vi "UHR-Fleezers Control (host) - 12.0_test_fpga_connection.vi"() -> ()   [LabVIEW 2014] (continued)
                n3308 = local read "N sets should be saved (MCL)"() -> (w5191:dbl)
                n3309 = Build Array(w5188, w5180, w5182, w5182, w5182) -> (w5186:dbl[])
                n3310 = Build Array(w5203, w5198, w5196, w5194, w5193, w5184, w5183) -> (w5200:dbl[])
                n3311 = Build Array(w5185, w5189, w5209, w5208, w5207, 3.0 ("t")) -> (w5202:dbl[])
                n3312 = Round Toward +Infinity(x=w5191) -> (ceil(x): smallest int >= x=w5192:dbl)
                n3313 = Build Array (concatenate)(w5202, w5201, w5186, w5200) -> (w5199:dbl[])
                n3314 = To Unsigned Long Integer(number=w5192) -> (unsigned 32bit integer=w5190:u32)
              }
            }
            n3315 = local read "Index"() -> (w5045:dbl)
            n3316 = call "Create new save file.vi"("Insert"="", "Ext"=".dat", "Index In"=w5045) -> ("Path Out"=w5004:path, "Index Out"=w5017:dbl)
            n3317 = local write "Save file name"(w5004) -> ()
            n3318 = local write "Index"(w5017) -> ()
            n3319 = local write "Save index"(w5017) -> ()
            n3320 = Array Size(array=w5028) -> (size(s)=w5029:i32)
            n3321 = Open/Create/Replace File(file path (use dialog)=w5004, operation (0:open)=T30."create", access (0:read/write)=enum16{"read/write", "read-only", "write-only"}."write-only") -> (refnum out=w5042:refnum<file>)  [unwired: 1 in, 4 out]
            n3322 = local write "Saving..."(TRUE ("Saving...")) -> ()
            n3323 = To Double Precision Float(number=w5029) -> (double precision float=w5027:dbl)
            n3324 = String Length(string="Comment (data description)") -> (length=w5025:i32)
            n3325 = To Double Precision Float(number=w5025) -> (double precision float=w5024:dbl)
            n3326 = Deny Access(7:w5042) -> (3:w5041:refnum<file>)  [unwired: 1 in, 2 out]
            n3327 = Build Array (concatenate)(w5027, w5028, w5024) -> (w5026:dbl[])
            n3328 = case "If fluorescence data to be saved" shown="True" w5015 {
              tunnel: w5004 -> [_ w5094]
              tunnel: [refnum<k0> refnum w5074] -> w5016
              frame False {
              }
              frame True {
                w5073 = 0.0
                n3329 = local read "APD Integration Time (s)"() -> (w5079:dbl)
                n3330 = local read "N APD Samp/step"() -> (w5072:dbl)
                n3331 = Path To String(path=w5094) -> (string=w5093:string)
                n3332 = String Length(string=w5093) -> (length=w5092:i32)
                n3333 = Subtract(x=w5092, y=4) -> (x-y=w5090:i32)
                n3334 = String Subset(string=w5093, length (rest)=w5090) -> (substring=w5089:string)  [unwired: 1 out]
                n3335 = Build Array(w5079, w5072, w5073, w5073, w5073, w5073, w5073, w5073) -> (w5076:dbl[])
                n3336 = Concatenate Strings(w5089, "_fl.dat" ("string")) -> (w5087:string)
                n3337 = Array Size(array=w5076) -> (size(s)=w5078:i32)
                n3338 = String To Path(string=w5087) -> (path=w5083:path)
                n3339 = Open/Create/Replace File(file path (use dialog)=w5083, operation (0:open)=T30."create", access (0:read/write)=enum16{"read/write", "read-only", "write-only"}."write-only") -> (refnum out=w5084:refnum<file>)  [unwired: 1 in, 4 out]
                n3340 = Deny Access(7:w5084) -> (3:w5080:refnum<file>)  [unwired: 1 in, 2 out]
                n3341 = To Double Precision Float(number=w5078) -> (double precision float=w5077:dbl)
                n3342 = Build Array (concatenate)(w5077, w5076) -> (w5075:dbl[])
                n3343 = Write to Binary File(file (use dialog)=w5080, data=w5075, 5:FALSE ("prepend array or string size? (T)"), 9:T29."big-endian, network order" ("byte order (0:big-endian, network order)")) -> (refnum out=w5074:refnum<file>)  [unwired: 1 in, 3 out]
              }
            }
            n3344 = case shown="True" w5002 {
              tunnel: w5004 -> [_ w5056]
              tunnel: [refnum<k0> refnum w5055] -> w5003
              frame False {
              }
              frame True {
                w5051 = 0.0 ("element")
                n3345 = Path To String(path=w5056) -> (string=w5070:string)
                n3346 = Build Array(w5051, w5051, w5051, w5051, w5051, w5051, w5051, w5051) -> (w5052:dbl[])
                n3347 = String Length(string=w5070) -> (length=w5069:i32)
                n3348 = Subtract(x=w5069, y=4) -> (x-y=w5067:i32)
                n3349 = Array Size(array=w5052) -> (size(s)=w5054:i32)
                n3350 = String Subset(string=w5070, length (rest)=w5067) -> (substring=w5066:string)  [unwired: 1 out]
                n3351 = To Double Precision Float(number=w5054) -> (double precision float=w5053:dbl)
                n3352 = Concatenate Strings(w5066, "_pos.dat" ("string")) -> (w5064:string)
                n3353 = Build Array (concatenate)(w5053, w5052) -> (w5050:dbl[])
                n3354 = String To Path(string=w5064) -> (path=w5060:path)
                n3355 = Open/Create/Replace File(file path (use dialog)=w5060, operation (0:open)=T30."create", access (0:read/write)=enum16{"read/write", "read-only", "write-only"}."write-only") -> (refnum out=w5061:refnum<file>)  [unwired: 1 in, 4 out]
                n3356 = Deny Access(7:w5061) -> (3:w5057:refnum<file>)  [unwired: 1 in, 2 out]
                n3357 = Write to Binary File(file (use dialog)=w5057, data=w5050, 5:FALSE ("prepend array or string size? (T)"), 9:T29."big-endian, network order" ("byte order (0:big-endian, network order)")) -> (refnum out=w5055:refnum<file>)  [unwired: 1 in, 3 out]
              }
            }
            n3358 = Write to Binary File(file (use dialog)=w5041, data=w5026, 5:w5022, 9:w5020) -> (refnum out=w5023:refnum<file>)  [unwired: 1 in, 3 out]
            n3359 = Write to Binary File(file (use dialog)=w5023, data="Comment (data description)", 5:w5022, 9:w5020) -> (refnum out=w5019:refnum<file>)  [unwired: 1 in, 3 out]
          }
        }
        n3360 = feedback-in #32(w4963) -> ()
        n3361 = feedback-in #33(w4989) -> ()
        n3362 = feedback-in #34(w4962) -> ()
        n3363 = feedback-in #35(w4973) -> ()
        n3364 = feedback-in #36(w4976) -> ()
        n3365 = feedback-in #37(w4988) -> ()
        n3366 = feedback-in #38(w4979) -> ()
      }
      frame #1 {
        n3367 = local read "Saving..."() -> (w5224:bool)
        n3368 = case shown="True" w5224 {
          tunnel: w5228 -> [_ w5240]
          tunnel: w5227 -> [_ w5253]
          tunnel: w5226 -> [_ w5249]
          tunnel: w5225 -> [_ w5248]
          tunnel: w5223 -> [_ w5229]
          tunnel: w5222 -> [_ w5243]
          tunnel: w5221 -> [_ w5242]
          tunnel: w5220 -> [_ w5241]
          tunnel: w5219 -> [_ w5239]
          tunnel: w5218 -> [_ w5237]
          tunnel: w5217 -> [_ w5236]
          tunnel: w5216 -> [_ w5235]
          tunnel: w5215 -> [_ w5234]
          tunnel: w5214 -> [_ w5233]
          tunnel: w5213 -> [_ w5232]
          tunnel: w5212 -> [_ w5231]
          tunnel: w5211 -> [_ w5230]
          frame False {
          }
          frame True {
            n3369 = Multiply(x=w5240, y=w5239) -> (x*y=→"Time (s)":dbl)
            n3370 = Less Or Equal?(x=w5240, y=w5229) -> (x <= y?=w5251:bool)
            n3371 = Or(x="Stop Saving", y="Abort save 2") -> (x .or. y?=w5244:bool)
            n3372 = Not(x=w5244) -> (.not. x?=w5252:bool)
            n3373 = And(x=w5251, y=w5252) -> (x .and. y?=w5250:bool)
            n3374 = case shown="True" w5250 {
              tunnel: w5253 -> [w5261 w5336]
              tunnel: [0.0 w5339] -> w5247
              tunnel: w5240 -> [_ w5337]
              tunnel: w5229 -> [_ w5338]
              tunnel: w5249 -> [_ w5333]
              tunnel: w5248 -> [_ _]
              tunnel: w5243 -> [w5259 w5326]
              tunnel: w5242 -> [w5258 w5327]
              tunnel: w5241 -> [_ w5325]
              tunnel: w5237 -> [_ w5324]
              tunnel: w5236 -> [_ w5268]
              tunnel: w5235 -> [_ w5317]
              tunnel: w5234 -> [_ w5295]
              tunnel: w5233 -> [w5255 w5277]
              tunnel: w5232 -> [w5256 w5276]
              tunnel: w5231 -> [_ w5273]
              tunnel: w5230 -> [_ w5271]
              frame False {
                w5257 = FALSE
                n3375 = Close File(refnum=w5261) -> ()  [unwired: 1 in, 2 out]
                n3376 = case shown="True" w5258 {
                  tunnel: w5259 -> [_ w5263]
                  frame False {
                  }
                  frame True {
                    n3377 = Close File(refnum=w5263) -> ()  [unwired: 1 in, 2 out]
                  }
                }
                n3378 = case shown="True" w5255 {
                  tunnel: w5256 -> [_ w5262]
                  frame False {
                  }
                  frame True {
                    n3379 = Close File(refnum=w5262) -> ()  [unwired: 1 in, 2 out]
                  }
                }
                n3380 = call <vilib>:"Beep.vi"() -> ()  [unwired: 3 in, 9 out]
                n3381 = local write "Raster Scanning..."(w5257) -> ()
                n3382 = local write "Calibrating..."(w5257) -> ()
                n3383 = property on="Abort wiggle" class="Bool (strict)"("Val(Sgnl)"=TRUE) -> ()  [unwired: 2 in, 2 out]
                n3384 = local write "Stop Saving"(w5257) -> ()
                "Saving..." <- w5257
              }
              frame True {
                n3385 = local read "Calibrating..."() -> (w5328:bool)
                n3386 = case "Write fl. data" shown="True" w5327 {
                  tunnel: w5326 -> [_ w5362]
                  tunnel: w5325 -> [_ w5361]
                  frame False {
                  }
                  frame True {
                    n3387 = Write to Binary File(file (use dialog)=w5362, data=w5361, 5:FALSE ("prepend array or string size? (T)"), 9:T29."big-endian, network order" ("byte order (0:big-endian, network order)")) -> ()  [unwired: 1 in, 4 out]
                  }
                }
                n3388 = Greater?(x="Save ave N", y=1.0) -> (0:w5331:bool)
                n3389 = Not(x=w5328) -> (.not. x?=w5330:bool)
                n3390 = And(x=w5330, y=w5331) -> (x .and. y?=w5274:bool)
                n3391 = case shown="True" w5274 {
                  tunnel: w5273 -> [w5342 w5353]
                  tunnel: [w5342 w5345] -> w5272
                  tunnel: "Save ave N" -> [_ w5346]
                  frame False {
                  }
                  frame True {
                    w5343 = 2 ("dimension size")
                    n3392 = Array Size(array=w5353) -> (size(s)=w5347:i32)
                    n3393 = Divide(x=w5347, y=w5343) -> (x/y=w5351:dbl)
                    n3394 = Reshape Array(w5353, w5351, w5343) -> (w5352:u64[][])
                    n3395 = Transpose 2D Array(2D array=w5352) -> (transposed array=w5350:u64[][])
                    n3396 = for {
                      tunnel: w5350 -> [w5355] mode=indexing
                      tunnel: [w5354] -> w5344 mode=indexing
                      tunnel: w5346 -> [w5356]
                      workers-P: _ -> [_]
                      n3397 = call "downsample 1D array - U64.vi"("Ave N"=w5356, "Array In"=w5355) -> ("Array Out"=w5354:u64[])  [unwired: 1 in]
                    }
                    n3398 = Transpose 2D Array(2D array=w5344) -> (transposed array=w5349:u64[][])
                    n3399 = Divide(x=w5347, y=w5346) -> (x/y=w5348:dbl)
                    n3400 = Reshape Array(w5349, w5348) -> (w5345:u64[])
                  }
                }
                n3401 = case shown="True" w5274 {
                  tunnel: w5333 -> [w5365 w5377]
                  tunnel: [w5365 w5369] -> w5329
                  tunnel: "Save ave N" -> [_ w5370]
                  tunnel: w5324 -> [_ w5368]
                  frame False {
                  }
                  frame True {
                    n3402 = Array Size(array=w5377) -> (size(s)=w5371:i32)
                    n3403 = Array Size(array=w5368) -> (size(s)=w5367:i32)
                    n3404 = Divide(x=w5371, y=w5367) -> (x/y=w5375:dbl)
                    n3405 = Reshape Array(w5377, w5375, w5367) -> (w5376:i16[][])
                    n3406 = Transpose 2D Array(2D array=w5376) -> (transposed array=w5374:i16[][])
                    n3407 = for {
                      tunnel: w5374 -> [w5380] mode=indexing
                      tunnel: [w5379] -> w5366 mode=indexing
                      tunnel: w5370 -> [w5378]
                      workers-P: _ -> [_]
                      n3408 = call "downsample 1D array - I16.vi"("Ave N"=w5378, "Array In"=w5380) -> ("Array Out"=w5379:i16[])  [unwired: 1 out]
                    }
                    n3409 = Transpose 2D Array(2D array=w5366) -> (transposed array=w5373:i16[][])
                    n3410 = Divide(x=w5371, y=w5370) -> (x/y=w5372:dbl)
                    n3411 = Reshape Array(w5373, w5372) -> (w5369:i16[])
                  }
                }
                n3412 = Index Array(array=w5295, index=1) -> (element=w5298:waveform(dbl))
                n3413 = Index Array(array=w5295, index=0) -> (element=w5300:waveform(dbl))
                n3414 = Unbundle By Name(w5298) -> ("Y"=w5302:dbl[])
                n3415 = Unbundle By Name(w5300) -> ("Y"=w5310:dbl[])
                n3416 = case "Write trap pos. data" shown="True" w5277 {
                  tunnel: w5276 -> [_ w5358]
                  tunnel: w5272 -> [_ w5357]
                  frame False {
                  }
                  frame True {
                    n3417 = Write to Binary File(file (use dialog)=w5358, data=w5357, 5:FALSE ("prepend array or string size? (T)"), 9:T29."big-endian, network order" ("byte order (0:big-endian, network order)")) -> ()  [unwired: 1 in, 4 out]
                  }
                }
                n3418 = Write to Binary File(file (use dialog)=w5336, data=w5329, 5:FALSE ("prepend array or string size? (T)"), 9:T29."big-endian, network order" ("byte order (0:big-endian, network order)")) -> ()  [unwired: 1 in, 4 out]
                n3419 = feedback #39(w5302) -> (w5304:dbl[])
                n3420 = Build Array (concatenate)(w5304, w5302) -> (w5303:dbl[])
                n3421 = Select(t=w5302, s=w5268, f=w5303) -> (s? t:f=w5288:dbl[])
                n3422 = feedback-in #39(w5288) -> ()
                n3423 = feedback #40(w5310) -> (w5323:dbl[])
                n3424 = Build Array (concatenate)(w5323, w5310) -> (w5322:dbl[])
                n3425 = Select(t=w5310, s=w5268, f=w5322) -> (s? t:f=w5297:dbl[])
                n3426 = feedback-in #40(w5297) -> ()
                n3427 = Divide(x=w5337, y=w5338) -> (x/y=w5340:dbl)
                n3428 = Multiply(x=w5340, y=100.0) -> (x*y=w5339:dbl)
                n3429 = Build Array(w5297, w5288) -> (→"Saved APD":dbl[][])
                n3430 = Array Size(array=w5297) -> (size(s)=w5315:i32)
                n3431 = Unbundle By Name(w5317) -> ("Y"=w5321:dbl[])
                n3432 = Subtract(x=w5315, y="N pts to average") -> (x-y=w5291:i32)
                n3433 = Multiply(x="N pts to average", y=u16 2) -> (x*y=w5292:u16)
                n3434 = Subtract(x=w5315, y=w5292) -> (x-y=w5290:i32)
                n3435 = feedback #41(w5321) -> (w5320:dbl[])
                n3436 = Build Array (concatenate)(w5320, w5321) -> (w5319:dbl[])
                n3437 = Select(t=w5321, s=w5268, f=w5319) -> (s? t:f=w5318:dbl[])
                "Trap Delta Graph" <- w5318
                n3438 = feedback-in #41(w5318) -> ()
                n3439 = Array Subset(array=w5297, index=w5291, length="N pts to average") -> (w5314:dbl[])
                n3440 = Array Subset(array=w5297, index=w5290, length="N pts to average") -> (w5313:dbl[])
                n3441 = Array Subset(array=w5288, index=w5291, length="N pts to average") -> (w5294:dbl[])
                n3442 = Array Subset(array=w5288, index=w5290, length="N pts to average") -> (w5293:dbl[])
                n3443 = Index Array(array=w5271, index=0) -> (element=w5269:waveform(dbl))
                n3444 = call-poly <vilib>:"Mean.vi"("X"=w5314) -> ("mean"=w5312:dbl)  [unwired: 1 out]
                n3445 = call-poly <vilib>:"Mean.vi"("X"=w5294) -> ("mean"=w5287:dbl)  [unwired: 1 out]
                n3446 = call-poly <vilib>:"Mean.vi"("X"=w5313) -> ("mean"=w5311:dbl)  [unwired: 1 out]
                n3447 = call-poly <vilib>:"Mean.vi"("X"=w5293) -> ("mean"=w5286:dbl)  [unwired: 1 out]
                n3448 = Unbundle By Name(w5269) -> ("Y"=w5266:dbl[])
                n3449 = Subtract(x=w5287, y=w5286) -> (x-y=w5278:dbl)
                "Delta Fl. 2" <- w5278
                n3450 = Subtract(x=w5312, y=w5311) -> (x-y=w5309:dbl)
                "Delta Fl. 1" <- w5309
                n3451 = Initialize Array(w5309, 1 ("dimension size")) -> (w5306:dbl[])
                n3452 = Initialize Array(w5278, 1 ("dimension size")) -> (w5283:dbl[])
                n3453 = feedback #42(w5306) -> (w5307:dbl[])
                n3454 = Build Array (concatenate)(w5307, w5306) -> (w5305:dbl[])
                n3455 = feedback #43(w5283) -> (w5284:dbl[])
                n3456 = Build Array (concatenate)(w5284, w5283) -> (w5282:dbl[])
                n3457 = feedback #44(w5266) -> (w5265:dbl[])
                n3458 = Build Array (concatenate)(w5265, w5266) -> (w5267:dbl[])
                n3459 = Select(t=w5266, s=w5268, f=w5267) -> (s? t:f=w5264:dbl[])
                "Saved trap pos" <- w5264
                n3460 = feedback-in #44(w5264) -> ()
                n3461 = Select(t=w5306, s=w5268, f=w5305) -> (s? t:f=w5281:dbl[])
                n3462 = feedback-in #42(w5281) -> ()
                n3463 = Select(t=w5283, s=w5268, f=w5282) -> (s? t:f=w5280:dbl[])
                n3464 = feedback-in #43(w5280) -> ()
                n3465 = Build Array(w5281, w5280) -> (→"Save APD Deriv":dbl[][])
              }
            }
            "Progress" <- w5247
            "Progress 2" <- w5247
          }
        }
      }
    }
    n3466 = local read "wait to reset values"() -> (w3911:bool)
    n3467 = Not(x=w3909) -> (.not. x?=w3912:bool)
    n3468 = And(x=w3912, y=w3911) -> (x .and. y?=w3913:bool)
    n3469 = case "Part of MCL raster scanning: returns to initial positions after scan done" shown="True" w3913 {
      tunnel: w3654 -> [w4782 w4789]
      tunnel: [w4782 w4788] -> w3915
      tunnel: w3653 -> [w4781 w4787]
      tunnel: [w4781 w4786] -> w3910
      frame False {
      }
      frame True {
        w4797 = 10.0 ("y")
        w4796 = 32767.0 ("y")
        # "to return scan values\nafter a synchronous \nAOM scan"
        n3470 = local read "AO2"() -> (w4790:dbl)
        n3471 = local read "AO1"() -> (w4791:dbl)
        n3472 = local write "wait to reset values"(FALSE ("wait to reset values")) -> ()
        n3473 = Multiply(x=w4791, y=w4796) -> (x*y=w4793:dbl)
        n3474 = Multiply(x=w4790, y=w4796) -> (x*y=w4795:dbl)
        n3475 = Divide(x=w4793, y=w4797) -> (x/y=w4792:dbl)
        n3476 = Divide(x=w4795, y=w4797) -> (x/y=w4794:dbl)
        n3477 = To Word Integer(number=w4792) -> (16bit integer=w4798:i16)
        n3478 = To Word Integer(number=w4794) -> (16bit integer=w4799:i16)
        n3479 = local read "Total Counts (ticks)"() -> (w4783:u32)
        n3480 = xnode "Read/Write Control"("FPGA VI Reference In"=w4789, "error in"=w4787, "AO1"=w4798, "AO2"=w4799, "MCL count"=w4783) -> ("FPGA VI Reference Out"=w4788:T22, "error out"=w4786:errorcluster)
        n3481 = local read "Scan Range (V)\n(of steps)"() -> (w4784:dbl)
        n3482 = property on="Scan Range (V)\n(of steps)" class="DigNum (strict)"("Val(Sgnl)"=w4784) -> ()  [unwired: 2 in, 2 out]
      }
    }
    n3483 = node-c288() -> ()  [unwired: 2 out]
  }
  n3484 = VISA Close(VISA resource name=w129, error in (no error)=w128) -> (error out=w172:errorcluster)
  n3485 = call <vilib>:"Simple Error Handler.vi"("error in (no error)"=w172) -> ()  [unwired: 1 in, 8 out]
  n3486 = node-c288(w134) -> ()  [unwired: 1 out]
  n3487 = node-c288(w216) -> ()  [unwired: 1 out]
  n3488 = flat-sequence {
    tunnel: w307 -> [w5384]
    tunnel: w309 -> [w5385]
    tunnel: [w5383] -> w289
    tunnel: [w5382] -> w288
    tunnel: w272 -> [_]
    tunnel: w224 -> [_]
    tunnel: w140 -> [_]
    tunnel: w289 -> [w5386]
    tunnel: w288 -> [w5387]
    frame #0 {
      w5381 = FALSE ("AI to FIFO")
      n3489 = xnode "Read/Write Control"("FPGA VI Reference In"=w5385, "error in"=w5384, "AI to FIFO"=w5381, "APD to FIFO"=w5381) -> ("FPGA VI Reference Out"=w5383:T22, "error out"=w5382:errorcluster)
    }
    frame #1 {
      n3490 = xnode "Close FPGA VI Reference"("FPGA VI Reference In"=w5386, "error in"=w5387) -> ("error out"=→"error out":errorcluster)
    }
  }
